vi "Keithley 6514 Measure Query.vi"(0 "Resource In":refnum<visa-resource-name>, 1 "Check For SCPI Errors? (T)":bool=TRUE, 5 "function (dc voltage:0)":u16(ring) items=["dc voltage", "dc current", "resistance", "charge"], 7 "Set Arm Count To 1? (F)":bool, 9 "Set Trig Count To 1? (F)":bool, 11 "error in (no error)":T1) -> (4 "Resource Out (dupl)":refnum<visa-resource-name>, 6 "Result":dbl, 15 "error out":T1)   [LabVIEW 2014, in "KE6514Driver.lvlib"]
doc: "The VI returns the result of a SCPI Signal Oriented MEASURE? command. This is equivalent to a one shot reading.\n\nThis is a basic VI for getting readings back and is not necessarily the best method but rather a quick way to getting measurements."
uses:
  KE6514Driver.lvlib
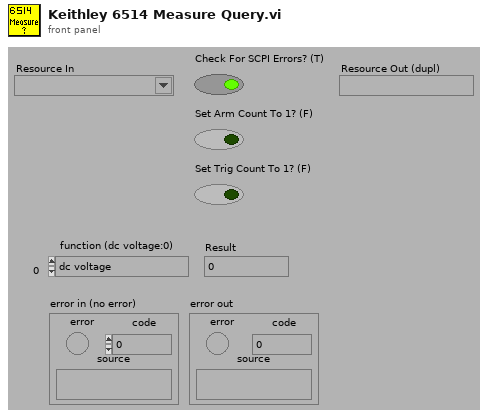
[diagram p1: front panel]
types:
  T1 = cluster{"error":bool, "code":i32, "source":string}
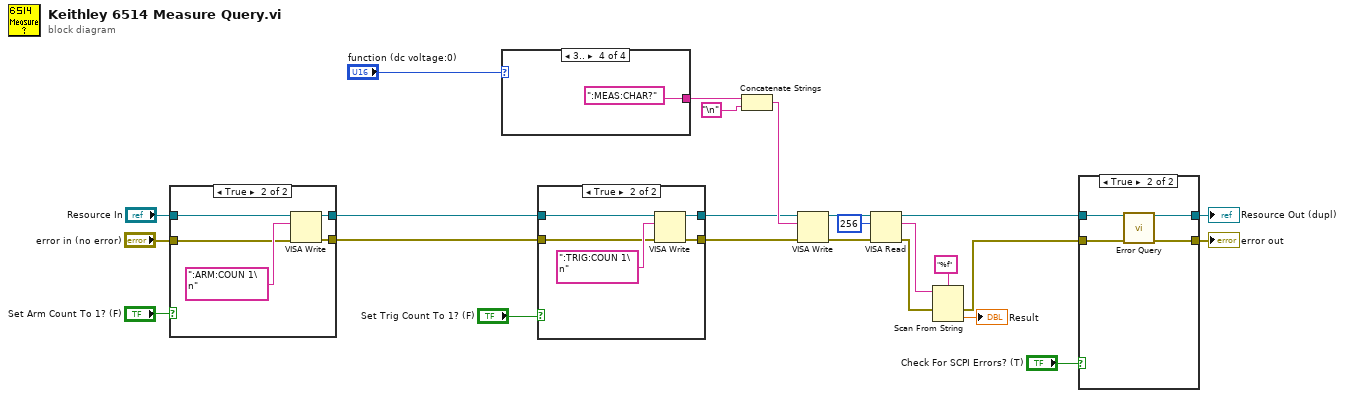
[diagram p0: block diagram]
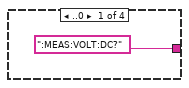
[diagram p5: hidden frame]
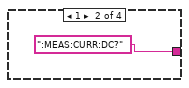
[diagram p6: hidden frame]
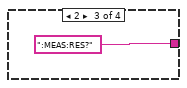
[diagram p7: hidden frame]
diagram:
  n1 = case shown="True" "Set Arm Count To 1? (F)" {
    tunnel: "Resource In" -> [w26 w30]
    tunnel: [w26 w29] -> w7
    tunnel: "error in (no error)" -> [w25 w28]
    tunnel: [w25 w27] -> w5
    frame False {
    }
    frame True {
      n2 = VISA Write(VISA resource name=w30, write buffer=":ARM:COUN 1\n", error in (no error)=w28) -> (VISA resource name out=w29:refnum<visa-resource-name>, error out=w27:errorcluster)  [unwired: 1 out]
    }
  }
  n3 = case "Selects Functions" shown="3.." "function (dc voltage:0)" {
    tunnel: [":MEAS:VOLT:DC?" ":MEAS:CURR:DC?" ":MEAS:RES?" ":MEAS:CHAR?"] -> w23
    frame ..0 {
    }
    frame 1 {
    }
    frame 2 {
    }
    frame 3.. {
    }
  }
  n4 = case shown="True" "Set Trig Count To 1? (F)" {
    tunnel: w7 -> [w37 w41]
    tunnel: w5 -> [w36 w40]
    tunnel: [w37 w39] -> w3
    tunnel: [w36 w38] -> w2
    frame False {
    }
    frame True {
      n5 = VISA Write(VISA resource name=w41, write buffer=":TRIG:COUN 1\n", error in (no error)=w40) -> (VISA resource name out=w39:refnum<visa-resource-name>, error out=w38:errorcluster)  [unwired: 1 out]
    }
  }
  n6 = Concatenate Strings(w23, "\n") -> (w21:string)
  n7 = VISA Write(VISA resource name=w3, write buffer=w21, error in (no error)=w2) -> (VISA resource name out=w20:refnum<visa-resource-name>, error out=w19:errorcluster)  [unwired: 1 out]
  n8 = VISA Read(VISA resource name=w20, byte count=u32 256, error in (no error)=w19) -> (VISA resource name out=w12:refnum<visa-resource-name>, read buffer=w17:string, error out=w14:errorcluster)  [unwired: 1 out]
  n9 = Scan From String(format string="%f", input string=w17, error in=w14) -> (error out=w11:errorcluster, output 1=→"Result":dbl)  [unwired: 2 in, 2 out]
  n10 = case shown="True" "Check For SCPI Errors? (T)" {
    tunnel: w12 -> [w44 w48]
    tunnel: w11 -> [w43 w47]
    tunnel: [w44 w46] -> w10
    tunnel: [w43 w45] -> w1
    frame False {
    }
    frame True {
      n11 = call "Error Query.vi"("VISA Resource In"=w48, "error in (no error)"=w47) -> ("VISA Resource Out (dupl)"=w46:refnum<visa-resource-name>, "error out"=w45:errorcluster)  [unwired: 10 in, 2 out]
    }
  }
  "Resource Out (dupl)" <- w10
  "error out" <- w1
